vi "Create HTML.vi"(8 "error in (no error)":errorcluster, 11 "Web FP In":refnum<class "Web Front Panel.lvclass">) -> (0 "error out":errorcluster, 2 "Created JS":path, 3 "Created HTML":path)   [LabVIEW 2015, in "Front Panel Publisher.lvlib" / "Front Panel Manager.lvclass"]
uses:
  Front Panel Manager.lvclass
  Web Front Panel_class/Web Front Panel.lvclass
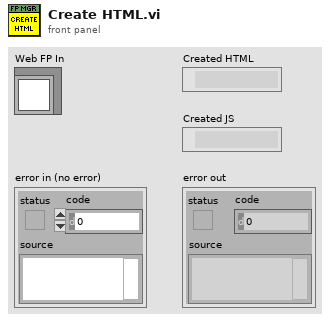
[diagram p1: front panel]
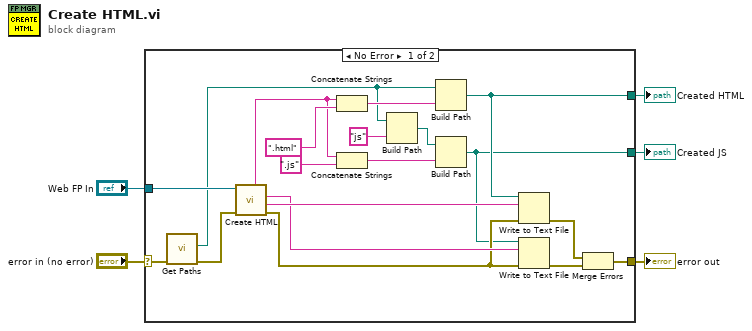
[diagram p0: block diagram]
diagram:
  n1 = case shown="No Error" "error in (no error)" {
    selector: "error in (no error)" -> [w9 w25]
    tunnel: [w13 w25] -> w4
    tunnel: "Web FP In" -> [w24 _]
    tunnel: [w7 _] -> w2
    tunnel: [w6 _] -> w1
    frame No Error {
      n2 = call "Get Paths.vi"("error in (no error)"=w9) -> ("error out"=w8:errorcluster, "Root folder"=w10:path)  [unwired: 7 in, 2 out]
      n3 = call-dynamic "Create HTML.vi"("error in (no error)"=w8, "Web FP In"=w24) -> ("error out"=w16:errorcluster, "HTML"=w18:string, "js"=w17:string, "Name"=w22:string)  [unwired: 5 in, 1 out]
      n4 = Concatenate Strings(w22, ".html") -> (w19:string)
      n5 = Concatenate Strings(w22, ".js") -> (w20:string)
      n6 = Build Path(base path=w10, name or relative path="js") -> (appended path=w11:path)
      n7 = Build Path(base path=w10, name or relative path=w19) -> (appended path=w7:path)
      n8 = Build Path(base path=w11, name or relative path=w20) -> (appended path=w6:path)
      n9 = Write to Text File(file (use dialog)=w7, text=w18, error in=w16) -> (error out=w14:errorcluster)  [unwired: 1 in, 2 out]
      n10 = Write to Text File(file (use dialog)=w6, text=w17, error in=w16) -> (error out=w15:errorcluster)  [unwired: 1 in, 2 out]
      n11 = Merge Errors(w14, w15) -> (w13:errorcluster)
    }
    frame Error {
    }
  }
  "error out" <- w4
  "Created HTML" <- w2
  "Created JS" <- w1
